vi "Get Exe Version.vi"(8 "error in (no error)":errorcluster, 11 "EXE Path (\"\")":path) -> (0 "error out":errorcluster, 1 "FileVersionInfo Out":T1, 2 "Version":T2 {"Build Date/Time" format="%<%X\n%x>T"})   [LabVIEW 2011]
uses:
  OGAB Version.ctl
  <vilib>/Platform/fileVersionInfo.llb/FileVersionInformation.ctl
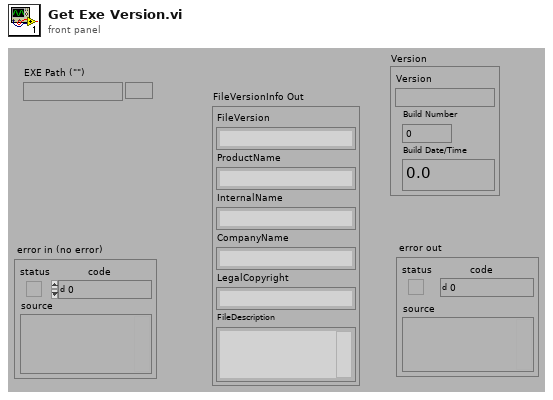
[diagram p1: front panel]
types:
  T1 = typedef "FileVersionInformation.ctl" = cluster{"FileVersion":string, "ProductName":string, "InternalName":string, "CompanyName":string, "LegalCopyright":string, "FileDescription":string}
  T2 = typedef "OGAB Version.ctl" = cluster{"Version":string, "Build Number":u32, "Build Date/Time":dbl}
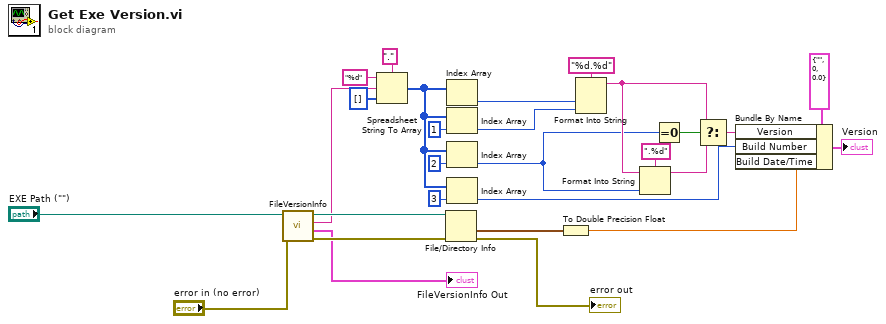
[diagram p0: block diagram]
diagram:
  n1 = call <vilib>:"FileVersionInfo.vi"("error in (no error)"="error in (no error)", "Application Path in"="EXE Path (\"\")") -> ("error out"=w18:errorcluster, "FileVersionInfo Out"=→"FileVersionInfo Out":T1, "File Version Info"=w15:string, "Application Path out"=w17:path)  [unwired: 6 out]
  n2 = Spreadsheet String To Array(delimiter (Tab)=".", format string="%d", spreadsheet string=w15, array type (2D Dbl)=i32[] []) -> (array=w6:i32[])
  n3 = File/Directory Info(path=w17, error in=w18) -> (last mod=w26:timestamp, error out=→"error out":errorcluster)  [unwired: 5 out]
  n4 = Index Array(array=w6) -> (element=w11:i32)  [unwired: 1 in]
  n5 = Index Array(array=w6, index=1) -> (element=w9:i32)
  n6 = Index Array(array=w6, index=2) -> (element=w7:i32)
  n7 = Index Array(array=w6, index=3) -> (element=w4:i32)
  n8 = To Double Precision Float(number=w26) -> (double precision float=w19:dbl)
  n9 = Format Into String(format string="%d.%d", w11, w9) -> (resulting string=w22:string)  [unwired: 2 in, 1 out]
  n10 = Format Into String(format string=".%d", initial string=w22, w7) -> (resulting string=w21:string)  [unwired: 1 in, 1 out]
  n11 = Equal To 0?(x=w7) -> (x = 0?=w25:bool)
  n12 = Select(t=w22, s=w25, f=w21) -> (s? t:f=w20:string)
  n13 = Bundle By Name(cluster=T2 {"Version"="", "Build Number"=0, "Build Date/Time"=0.0} ("Version"), "Version"=w20, "Build Number"=w4, "Build Date/Time"=w19) -> (→"Version":T2)
